vi "Manual CE-CERT Inverter MODBUS TCP-IP Read-Write Registers.vi"() -> ()   [LabVIEW 2018]
uses:
  <vilib>/Plasmionique/MB Master/MB_Master_TCP/MB_Master_TCP.lvclass
  C:/Program Files (x86)/National Instruments/LabVIEW 2018/vi.lib/Plasmionique/MB Master/MB_Master/MB_Master.lvclass
  <vilib>/Plasmionique/MB Master/MB Master.lvlib
panel:
  in  "Read Two Registers (SGL) Starting Address":u16
  out "Read Two U16 Registers (SGL)":sgl
  in  "Write Holding Register Value":u16
  in  "Write Holding Register Address":u16
  in  "Read Single Holding Register Address":u16=29
  in  "IP Address":string
  in  "Write Holding Register":bool
  out "Read Single Input Register Value":u16
  in  "Read Single Input Register Address":u16
  in  "Stop Program":bool
  out "Read Single Holding Register Value":u16
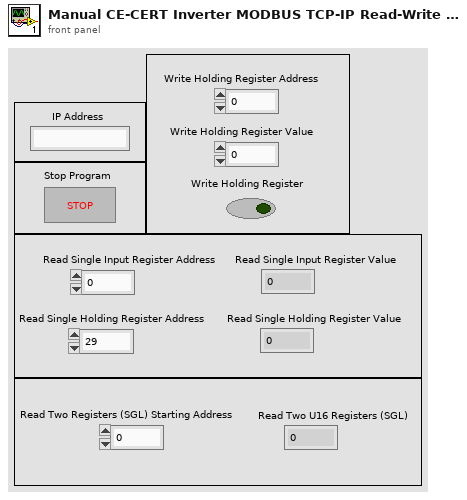
[diagram p1: front panel]
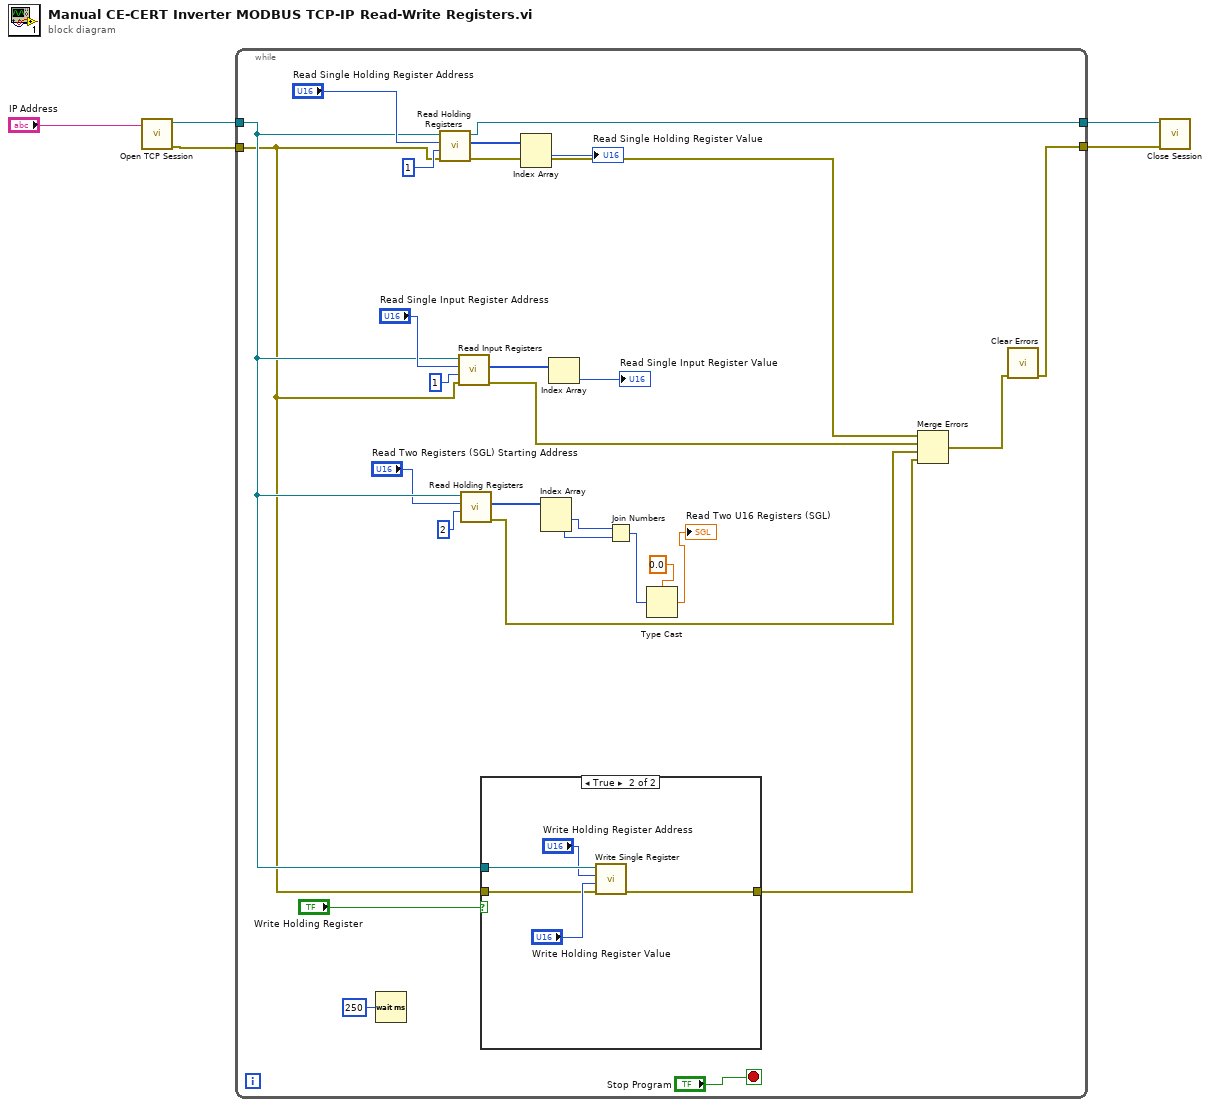
[diagram p0: block diagram]
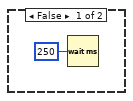
[diagram p2: hidden frame]
diagram:
  n1 = call <vilib>:"Open TCP Session.vi"("IP Address"="IP Address") -> ("error out"=w2:errorcluster, "MB_TCP session"=w4:refnum<class "MB_Master_TCP.lvclass">)  [unwired: 9 in]
  n2 = while {
    tunnel: w4 -> [w20]
    tunnel: [w22] -> w5
    tunnel: w2 -> [w12]
    tunnel: [w10] -> w1
    stop <- "Stop Program" stop-if-true
    n3 = Wait (ms)(milliseconds to wait=u32 250) -> ()  [unwired: 1 out]
    n4 = call <vilib>:"Read Holding Registers.vi"("error in (no error)"=w12, "quantity"=u16 1, "starting address"="Read Single Holding Register Address", "MB session in"=w20) -> ("error out"=w9:errorcluster, "Registers"=w27:u16[], "MB session out"=w22:refnum<class "MB_Master_TCP.lvclass">)  [unwired: 5 in]
    n5 = call <vilib>:"Read Input Registers.vi"("error in (no error)"=w12, "quantity"=u16 1, "starting address"="Read Single Input Register Address", "MB session in"=w20) -> ("error out"=w8:errorcluster, "Registers"=w30:u16[])  [unwired: 5 in, 1 out]
    n6 = call <vilib>:"Read Holding Registers.vi"("quantity"=u16 2, "starting address"="Read Two Registers (SGL) Starting Address", "MB session in"=w20) -> ("error out"=w7:errorcluster, "Registers"=w19:u16[])  [unwired: 6 in, 1 out]
    n7 = case shown="True" "Write Holding Register" {
      tunnel: w20 -> [_ w39]
      tunnel: w12 -> [_ w36]
      tunnel: [_ w35] -> w6
      frame False {
        n8 = Wait (ms)(milliseconds to wait=u32 250) -> ()  [unwired: 1 out]
      }
      frame True {
        n9 = call <vilib>:"Write Single Register.vi"("error in (no error)"=w36, "value"="Write Holding Register Value", "address"="Write Holding Register Address", "MB session in"=w39) -> ("error out"=w35:errorcluster)  [unwired: 6 in, 1 out]
      }
    }
    n10 = Index Array(array=w27) -> (element #1=→"Read Single Holding Register Value":u16)  [unwired: 2 in, 1 out]
    n11 = Index Array(array=w19) -> (element #1=w18:u16, element #2=w17:u16)  [unwired: 2 in]
    n12 = Index Array(array=w30) -> (element=→"Read Single Input Register Value":u16)  [unwired: 1 in]
    n13 = Join Numbers(hi=w18, lo=w17) -> ((hi.lo)=w15:u32)
    n14 = Type Cast(type=sgl 0.0, x=w15) -> (*(type *) &x=→"Read Two U16 Registers (SGL)":sgl)
    n15 = Merge Errors(w9, w8, w7, w6) -> (w11:errorcluster)
    n16 = call <vilib>:"Clear Errors.vi"("error in (no error)"=w11) -> ("error out"=w10:errorcluster)  [unwired: 5 in, 1 out]
  }
  n17 = call-dynamic "Close Session.vi"("error in (no error)"=w1, "MB TCP session"=w5) -> ()  [unwired: 9 in, 1 out]
